vi "SYST_PRES.vi"(0 "VISA IN":refnum<visa-resource-name>, 5 "error in":errorcluster) -> (14 "VISA Out":refnum<visa-resource-name>, 19 "error out":errorcluster)   [LabVIEW 2018, in "PNA-X.lvlib"] (continued)
DISPlay:WINDow<wnum>:TRACe<tnum>TITLe:DATA? \nReturn Type String \nDefault Not Applicable \nDISPlay:WINDow<wnum>:TRACe<tnum>TITLe:STATe <bool> \n(Read-Write) Turns display of the Trace Title ON or OFF. When turned OFF, the previous trace title \nreturns. Set a new trace title using DISP:WIND:TRAC:TITL:DATA \nLearn more about Trace Titles \nParameters \n<wnum> Any existing window number. If unspecified, value is set to 1 \n<tnum> Trace number of the specified window. If unspecified, value is set to 1. The \ntrace number displayed in trace status is the trace number of the channel; not \nthe window. Use Display:Cat? to read the window numbers. Use \nDisp:Window:Cat? to read the trace numbers of the specified window. \n<bool> ON (or 1) - turns the title ON. \nOFF (or 0) - turns the title OFF. \nExamples DISP:WIND:TRAC:TITL ON \nDisplay:window2:trace3:title:state off \nQuery Syntax DISPlay:WINDow<wnum>:TRACe<tnum>:TITLe[:STATe]? \n1598\n\nReturn Type Boolean (1 = ON, 0 = OFF) \nDefault ON \nDISPlay:WINDow<wnum>:TRACe<tnum>:Y[:SCALe]:AUTO \n(Write-only) Performs an Autoscale on the specified trace in the specified window, providing the best \nfit display. Autoscale is performed only when the command is sent; it does NOT keep the trace \nautoscaled indefinitely. \nParameters \n<wnum> Any existing window number. If unspecified, value is set to 1. \n<tnum> Any existing trace number; if unspecified, value is set to 1 \nExamples DISP:WIND:TRAC:Y:AUTO \ndisplay:window2:trace2:y:scale:auto \nQuery Syntax Not applicable \nDefault Not applicable \nDISPlay:WINDow<wnum>:TRACe<tnum>:Y[:SCALe]:PDIVision <num> \n(Read-Write) Sets the Y axis Per Division value of the specified trace in the specified window. \nParameters \n<wnum> Any existing window number. If unspecified, value is set to 1. \n<tnum> Any existing trace number; if unspecified, value is set to 1 \n<num> Units / division value. The range of acceptable values is dependent on format \nand domain. \nNote: This command will accept MIN or MAX instead of a numeric \nparameter. See SCPI Syntax for more information. \nExamples DISP:WIND:TRAC:Y:PDIV 1 \ndisplay:window2:trace2:y:scale:pdivision maximum \nQuery Syntax DISPlay:WINDow<wnum>:TRACe<tnum>:Y[:SCALe]:PDIVision? \nReturn Type Numeric \nDefault 10 \nDISPlay:WINDow<wnum>:TRACe<tnum>:Y[:SCALe]:RLEVel <num> \n1599\n\n(Read-Write) Sets the Y axis Reference Level of the specified trace in the specified window. \nParameters \n<wnum> Any existing window number. If unspecified, value is set to 1. \n<tnum> Any existing trace number; if unspecified, value is set to 1 \n<num> Reference level value. The range of acceptable values is dependent on format \nand domain. \nNote: This command will accept MIN or MAX instead of a numeric parameter. \nSee SCPI Syntax for more information. \nExamples DISP:WIND:TRAC:Y:RLEV 0 \ndisplay:window2:trace2:y:scale:rlevel minimum \nQuery Syntax DISPlay:WINDow<wnum>:TRACe<tnum>:Y[:SCALe]:RLEVel? \nReturn Type Numeric \nDefault NA \nDISPlay:WINDow<wnum>:TRACe<tnum>:Y[:SCALe]:RPOSition <num> \n(Read-Write) Sets the Reference Position of the specified trace in the specified window \nParameters \n<wnum> Any existing window number. If unspecified, value is set to 1. \n<tnum> Any existing trace number; if unspecified, value is set to 1 \n<num> Reference position on the screen measured in horizontal graticules from the \nbottom. The range of acceptable values is dependent on format and domain. \nNote: This command will accept MIN or MAX instead of a numeric \nparameter. See SCPI Syntax for more information. \nExamples DISP:WIND:TRAC:Y:RPOS 0 \ndisplay:window2:trace2:y:rposition maximum \nQuery Syntax DISPlay:WINDow<wnum>:TRACe<tnum>:Y[:SCALe]:RPOSition? \nReturn Type Numeric \nDefault 5 \nDISPlay:VISible <ON | OFF> \n1600\n\n(Read-Write) Makes the PNA application visible or not visible. In the Not Visible state, the analyzer \ncycle time for making measurements, and especially data transfer, can be significantly faster because \nthe display does not process data. \nParameters \n<ON | OFF> ON (or 1) - PNA app is visible \nOFF (or 0) - PNA app is NOT visible \nExamples DISP:VIS ON \ndisplay:visible off \nQuery Syntax DISPlay:VISible? \nReturn Type Boolean (1 = ON, 0 = OFF) \nDefault ON \nLast modified: \n9/12/06 Modified for number of windows. \n1601\n\nFormat Commands \nSpecifies the way that data will be transferred when moving large amounts of data. These commands \nwill affect data that is transferred with the CALC:DATA and CALC:RDATA commands. \nClick on a blue keyword to view the command details. \nSee Also \nExample Programs \nSynchronizing the PNA and Controller \nSCPI Command Tree \nFORMat:BORDer <char> \n(Read-Write) Set the byte order used for GPIB data transfer. Some computers read data from the \nanalyzer in the reverse order. This command is only implemented if FORMAT:DATA is set to \n:REAL. If FORMAT:DATA is set to :ASCII, the swapped command is ignored. \nParameters \n<char> Choose from: \nNORMal - Use when your controller is anything other than an IBM compatible \ncomputers \nSWAPped - for IBM compatible computers \nNote: Use NORMal if you are using drivers like VISA or development \nenvironments like VEE, LabView, or T&M Tool kit. \nExamples FORM:BORD SWAP \nformat:border normal \nQuery Syntax FORMat:BORDer? \nReturn Type Character \n1602\n\nDefault Normal \nFORMat[:DATA] <char> \n(Read-Write) Sets the data format for data transfers. \nTo transfer measurement data, use CALC:DATA. \nTo transfer Cal Set data, use \nTo transfer Source Power correction data, use \nSOURce:POWer:CORRection:COLLect:TABLe:DATA \nSOURce:POWer:CORRection:COLLect:TABLe:FREQuency \nSOURce:POWer:CORRection:DATA \nParameters \n<char> Choose from: \nREAL,32 - (default value for REAL) Best for transferring large amounts of \nmeasurement data. \nREAL,64 - Slower but has more significant digits than REAL,32. Use \nREAL,64 if you have a computer that doesn't support REAL,32. \nASCii,0 - The easiest to implement, but very slow. Use if small amounts of \ndata to transfer. \nNote: The REAL,32 and REAL,64 arguments transfer data in block format as \nexplained in Transferring Measurement Data. \nExamples FORM REAL,64 \nformat:data ascii \nQuery Syntax FORMat:DATA? \nReturn Type Character,Character \nDefault ASCii,0 \n1603\n\nHardcopy Command \nLearn about Printing \nSCPI Command Tree \nHCOPy:FILE <filename> \n(Write-only) Saves the screen image to a file. \nParameters \n<filename> Name of the file to save the screen to. The file is saved to the current working \ndirectory unless a valid full path name is specified. \nUse one of the following suffixes: \n.bmp - not recommended due to large file size \n.jpg - not recommended due to poor quality \n.png - recommended \nExamples HCOPY:FILE \"myFile.png\" \nhcopy:file \"c:\\data\\myfile.png\" \nQuery Syntax Not Applicable \nDefault Not Applicable \nHCOPy[:IMMediate] \n(Write-only) Prints the screen to the default printer. \nExamples HCOP \nhcopy:immediate \nQuery Syntax Not applicable \nDefault Not Applicable \n1604\n\nInitiate Commands \nControls triggering signals \nClick on a blue keyword to view the command details. \nSee Also \nExample Triggering the PNA \nLearn about Triggering \nSynchronizing the PNA and Controller \nSCPI Command Tree \nINITiate:CONTinuous <boolean> \n(Read-Write) Specifies whether the PNA trigger source is set to Internal (continuous) or Manual. \nThis command is a subset of TRIG:SEQ:SOURce, which can also set the trigger source to External. \nTo set how a channel responds to trigger signals, use SENS:SWE:MODE. \nSee a map of user interface to SCPI triggering commands. \nFor more information on triggering, see the PNA Trigger Model. \nSee the Example program: Triggering the PNA using SCPI. \nParameters \n<boolean> ON (or 1) - Internal (continuous) trigger. \nOFF (or 0) - Manual sweep. Use INIT:IMMediate to send a trigger signal \nExamples INIT:CONT ON \ninitiate:continuous off \nQuery Syntax INITiate:CONTinuous? \nReturn Type Boolean (1 = ON, 0 = OFF) \nDefault ON \n1605\n\nINITiate<cnum>[:IMMediate] \n(Write-only) Stops the current sweeps and immediately sends a trigger. (Same as Trigger! on the PNA \nfront panel). \nSee the Example program: Triggering the PNA using SCPI \nNote: An SMC Fixed Output measurement cannot be triggered using this command. For more \ninformation, see the example program. \nThis command requires Trigger:Source to be set to Manual. This causes ONE trigger signal to be \nSENT each time INIT:IMM is issued. \nSens<ch>:Sweep:Mode sets the number of trigger signals each channel will ACCEPT (Continuous - \nunlimited, Groups - a specific number, or HOLD - none.) \nTo trigger ALL channels in turn: \nSet ALL channels to Sens<ch>:Sweep:Mode Continuous. The <ch> argument in INIT<ch>:IMM is \nignored. \nThen�\nTRIG:SCOP ALL triggers ALL channels (in sequence) each time Init:Imm is sent. \nTRIG:SCOP CURRent triggers ONLY the NEXT channel each time Init:Imm is sent. \nTo trigger ONLY a specified channel: \nSet ALL channels to Sens<ch>:Sweep:Mode HOLD 1. \nSend TRIG:SCOP CURRent 2. \nSend Init<ch>:Imm where <ch> is the channel to be triggered. 3. \nAdvanced Situations that require some channels to be in CONT and others in HOLD are rare. The \nfollowing describes the behavior of the Init:Imm command in these situations: \nWhen Trigger:Scope = Global: \nIf the SPECIFIED <cnum> channel is in hold mode, it is put in single trigger (accepts 1 trigger signal) and \ngoes to the end of the queue of channels to be triggered. The other 'non-hold' channels are triggered. The \nnext Init:Imm triggers the specified channel first. \nFor example: ch1 is in Hold, ch2 and ch3 are in CONT and we send INIT1:IMM \n1606\n\nOn the first INIT:IMM, ch2 and ch3 is triggered. \nnext INIT:IMM, ch1, ch2, ch3 is triggered. \nnext INIT:IMM, ch2 and ch3 is triggered. \nnext INIT:IMM, ch1, ch2, ch3 is triggered, and so forth. \nWhen Trigger:Scope = Channel \nOnly ONE channel is triggered for each issued INIT<ch>:IMM command. \nIf the specified channel is in hold, it is put in single trigger (accepts 1 trigger signal) and goes the end of the \nqueue of channels to be triggered as in the 'Global' example. \nThis is one of the PNA overlapped commands. Learn more. \nParameters \n<cnum> Any existing channel number. If unspecified, value is set to 1 \nExamples INIT \ninitiate2:immediate \nQuery Syntax Not applicable \nDefault Not applicable \nLast modified: \nApril 23, 2007 Updated Init:Imm \n1607\n\nMemory Commands \nThe memory commands control saving and loading instrument states and measurement trace data to the \nhard drive. To read and write trace data in GPIB format, see CALC:DATA. \nClick on a blue keyword to view the command details. \nSee Also \nExample Programs \nLearn about Save / Recall and File Types \nSynchronizing the PNA and Controller \nSCPI Command Tree \nSpecifying Path Names \nThe MMEM commands use the following rules to specify path names: \nThe default folder is \"C:\\Program Files\\Agilent\\Network Analyzer\\Documents\" \nYou can change the active directory using MMEMory:CDIRectory. \nSpecify only the file name if using the active directory. \nYou can also use an absolute path name to specify the folder and file. \nMMEMory:CATalog[:<char>]? [<folder>] \n1608\n\n(Read-only) Returns a comma-separated string of file names that are in the specified folder. If there \nare no files of the specified type, \"NO CATALOG\" is returned. Learn about File Types \nParameters \n<char> The type of files to list. Choose from: \nSTATe - Instrument states (.sta) \nCORRection - Calibration Data (.cal) \nCSARchive - Instrument state and calibration data (.csa) \nCSTate - Instrument state and link to Calibration data (.cst) \nIf unspecified then ALL file types (even unknown types) are listed. \n<folder> String - Any existing folder name. See Specifying Path Names \nExamples MMEM:CAT? 'lists all files from the current folder \nmmemory:catalog:correction? 'C:\\Program Files\\Agilent\\Network \nAnalyzer\\Documents' 'lists .cal files from the specified folder \nDefault Not applicable \nMMEMory:CDIRectory <folder> \n(Read-Write) Changes the folder name. \nParameters \n<folder> Any drive and folder name that already exists. \nIf the same level as \"C:\\Program Files\\Agilent\\Network Analyzer\\Documents\", \nthen no punctuation is required \nMMEM:CDIR Service \nIf the new folder is at a different level than \"C:\\Program Files\\Agilent\\Network \nAnalyzer\\Documents\", use a slash (\\) before the folder name and enclose in \nquotes. \nmmemory:cdirectory '\\automation' 'changes default directory up \none level. \nYou can use an absolute path to specify the new folder. \nmmemory:cdirectory 'c:\\automation\\service' \nQuery Syntax MMEMory:CDIRectory? 'Returns the current folder name \n1609\n\nReturn Type String \nDefault 'C:\\Program Files\\Agilent\\Network Analyzer\\Documents' \nMMEMory:COPY <file1>,<file2> \n(Write-only) Copies file1 to file2. Extensions must be specified. \nParameters \n<file1> String - Name of the file to be copied. See Specifying Path Names \n<file2> String - Name of the file to be created from file1. \nExamples MMEM:COPY 'MyFile.cst','YourFile.cst' \nQuery Syntax Not applicable \nDefault Not applicable \nMMEMory:DELete <file> \n(Write-only) Deletes file. Extensions must be specified. \nParameters \n<file> String - Name of the file to be deleted. See Specifying Path Names \nExamples MMEM:DEL 'MyFile.cst' \nQuery Syntax Not applicable \nDefault Not applicable \nMMEMory:LOAD[:<char>] <file> \n1610\n\n(Write-only) Loads the specified file. Learn about File Types \nParameters \n<char> The type of file to load. Choose from: \nSTATe - Instrument states (.sta) \nCORRection - Calibration Data (.cal) \nCSARchive - Instrument state and calibration data (.csa) \nCSTate - Instrument state and link to Calibration data (.cst) \nIf <char> is unspecified, the extension must be included in the filename. \nIf an extension is specified in <file> that does not agree with <char> then no \naction is taken. \n<file> String - Name of the file to be loaded. See Specifying Path Names \nExamples MMEM:LOAD 'MyFile.cst' \nmmemory:load:state 'MyInstState' \nQuery Syntax Not applicable \nDefault Not applicable \nMMEMory:MDIRectory <folder> \n(Write-only) Makes a folder. \nParameters \n<folder> String - Name of the folder to make. See Specifying Path Names \nExamples MMEM:MDIR 'MyFolder' \nmmemory:mdirectory 'c:\\NewFolder' \nQuery Syntax Not applicable \nDefault Not applicable \nMMEMory:MOVE <file1>,<file2> \n1611\n\n(Write-only) Renames <file1> to <file2>. File extensions must be specified. \nParameters \n<file1> String - Name of the file to be renamed. See Specifying Path Names \n<file2> String - Name of the new file. \nExamples MMEM:MOVE 'MyFile.cst','YourFile.cst' \nQuery Syntax Not applicable \nDefault Not applicable \nMMEMory:RDIRectory <folder> \n(Write-only) Removes the specified folder. \nParameters \n<folder> String - Name of the folder to remove. See Specifying Path Names \nExamples MMEM:RDIR 'MyFolder' \nQuery Syntax Not applicable \nDefault Not applicable \nMMEMory:STORe[:<char>] <file> \n(Write-only) Stores the specified file (.sta, .cal, .csa, .cst, prn). \nTo save snp files, use Calc:Data:SNP:PORTs:SAVE. \nTo save *.cti files, use MMEM:STOR:CIT:DATA or MMEM:STOR:CIT:FORM. \nParameters \n<char> The type of file to store. Choose from: \nSTATe - Instrument states (.sta) \nCORRection - Calibration Data (.cal) \nCSARchive - Instrument state and calibration data (.csa) \nCSTate - Instrument state and link to Calibration data (.cst) \nNo <char> is specified for prn. \n1612\n\nIf <char> is unspecified, then the extension must be included in the filename. \nIf an extension is specified in <file> that does not agree with <char> then no \naction is taken. \nLearn about File Types \n<file> String - Name of any valid file that is not already in existence. See Specifying \nPath Names \nExamples MMEM:STOR:STAT 'myState' \nmmemory:store 'c:\\bin\\myState.sta' \nMMEM:STOR 'MyData.prn' \nQuery Syntax Not applicable \nDefault Not applicable \nMMEMory:STORe:CITifile:DATA <filename> \n(Write only) Saves UNFORMATTED trace data to .cti file. Learn more. \nParameters \n<filename> Any drive and folder name that already exists. \nIf the same level as \"C:\\Program Files\\Agilent\\Network Analyzer\\Documents\", \nthen no punctuation is required \nMMEM:STOR:CIT:DATA MYCTIFile \nIf the new folder is at a different level than \"C:\\Program Files\\Agilent\\Network \nAnalyzer\\Documents\", use a slash (\\) before the folder name and enclose in \nquotes. \nmmemory:cdirectory '\\automation' 'changes default directory up \none level. \nYou can use an absolute path to specify the new folder. \nmmemory:cdirectory 'c:\\automation\\service' \nQuery Syntax Not Applicable \nDefault C:\\Program Files\\Agilent\\Network Analyzer\\Documents' \nMMEMory:STORe:CITifile:FORMat <filename> \n1613\n\n(Write only) Saves FORMATTED trace data to .cti file. Learn more. \nParameters \n<filename> Any drive and folder name that already exists. \nIf the same level as \"C:\\Program Files\\Agilent\\Network Analyzer\\Documents\", \nthen no punctuation is required \nMMEM:STOR:CIT:DATA MYFile \nIf the new folder is at a different level than \"C:\\Program Files\\Agilent\\Network \nAnalyzer\\Documents\", use a slash (\\) before the folder name and enclose in \nquotes. \nmmemory:cdirectory '\\automation' 'changes default directory up \none level. \nYou can use an absolute path to specify the new folder. \nmmemory:cdirectory 'c:\\automation\\service' \nQuery Syntax Not Applicable \nDefault C:\\Program Files\\Agilent\\Network Analyzer\\Documents' \nMMEMory:STORe:TRACe:CONTents:CITifile <char> \n(Read-Write) Specifies the contents of subsequent citifile save statements. (See Data Define Saves) \nParameters \n<char> Choose from: \nSING - Single trace \nDISP - All displayed traces \nAUTO - All displayed traces \nExamples MMEM:STOR:TRAC:CONT:CIT SING \nQuery Syntax MMEMory:STORe:TRACe:CONTents? \nReturn Type Character \nDefault Auto \nMMEMory:STORe:TRACe:FORMat:CITifile <char> \n1614\n\n(Read-Write) Specifies the format of subsequent citifile save statements. (See Data Define Saves) \nParameters \n<char> Format in which the citifile will be saved with subsequent \nMMEMory:STORe:CIT:FORMat statements. Choose from: \nMA - Linear Magnitude / degrees \nDB - Log Magnitude / degrees \nRI - Real / Imaginary \nAUTO - Format in which the trace is already displayed. If other than Log \nMag, Linear Magnitude, or Real/Imag, then the format will be in Real/Imag. \nExamples MMEM:STOR:TRAC:FORM:CIT MA \nQuery Syntax MMEMory:STORe:TRACe:FORMat:CITifile? \nReturn Type Character \nDefault Auto' \nMMEMory:STORe:TRACe:FORMat:SNP <char> \n(Read-Write) Specifies the format of subsequent .s1p, .s2p, .s3p; s4p save statements. (See Data \nDefine Saves). \nParameters \n<char> Choose from: \nMA - Linear Magnitude / degrees \nDB - Log Magnitude / degrees \nRI - Real / Imaginary \nAUTO - data is output in currently selected trace format. If other than LogMag, \nLinMag, or Real/Imag, then output is in Real/Imag. \nExamples MMEM:STOR:TRAC:FORM:SNP MA \nQuery Syntax MMEMory:STORe:TRACe:FORMat:SNP? \nReturn Type Character \nDefault Auto' \n1615\n\nMMEMory:TRANsfer <fileName>,<dataBlock> \n(Read-Write) Transfers data between the PNA and an external controller. Other MMEM commands \ntransfer data between the PNA application and the PNA hard drive. If <fileName> already exists, it \nwill be overwritten. The file must be no larger than 20MB. \nTo read trace data from the PNA in block format, use CALC:DATA. \nParameters \n<fileName> String - File name. See Specifying Path Names \n<dataBlock> Block Data - The contents of the file. \nThe data block is a block of binary data. Use the following syntax: \n#<num digits><byte count><data bytes><NL><END> \nwhere: \n<num_digits> specifies how many digits are contained in <byte_count> \n<byte_count> specifies how many data bytes will follow in <data bytes> \nExample See example program \nQuery Syntax MMEMory:TRANsfer? <fileName> \nReads block data from the specified file location. \nDefault Not applicable \nLast modified: \n9/12/06 MQ Store command has reference to PORTS Snp. \n1616\n\nOutput Command \nLearn about Power \nOUTPut[:STATe] <ON | OFF> \n(Read-Write) Turns RF power from the source ON or OFF. \nSee note about source power state with instrument state save and recall. \nParameters \n<ON | OFF> ON (or 1) - turns RF power ON \nOFF (or 0) - turns RF power OFF \nExamples OUTP ON \noutput:state off \nQuery Syntax OUTPut[:STATe]? \nReturn Type Boolean (1 = ON, 0 = OFF) \nDefault ON \n1617\n\nRoute Command \nLearn about Frequency Offset \nSCPI Command Tree \nROUTe<cnum>:PATH:LOOP[:R1] <char> \n(Read-Write) Throws internal switch to reference receiver when the specified channel is measured. \nThis feature is only available on PNA models with Option 081 - external reference switch. See block \ndiagram of the reference switch. \nParameters \n<cnum> Any existing channel number. If unspecified, value is set to 1 \n<char> Position of the switch. Choose from: \nINTernal - bypass R1 Loop. Connects the port 1 source directly to the R1 \nreceiver. \nEXTernal - flow through R1 Loop. Allows direct access to the R1 receiver \nthrough the Reference 1 front-panel connectors. \nExamples ROUT:PATH:LOOP INT \nroute2:path:loop:r1 external \nQuery Syntax ROUTe<cnum>:PATH:LOOP:R1? \nReturn Type Character \nDefault INTernal \n1618\n\nSense:Average Commands \nSets sweep-to-sweep averaging parameters. Averaging is a noise reduction technique that averages \neach data point over a user-specified number of sweeps. Averaging affects all of the measurements in \nthe channel. \nClick on a blue keyword to view the command details. \nSee Also \nExample using some of these commands. \nLearn about Averaging \nSynchronizing the PNA and Controller \nSCPI Command Tree \nSENSe<cnum>:AVERage:CLEar \n(Write-only) Clears and restarts averaging of the measurement data. Must also set \nSENS:AVER[:STATe] ON \nParameters \n<cnum> Any existing channel number; if unspecified, value is set to 1. \nExamples SENS:AVER:CLE \nsense2:average:clear \nQuery Syntax Not applicable \nDefault Not applicable \nSENSe<cnum>:AVERage:COUNt <num> \n1619\n\n(Read-Write) Sets the number of measurement sweeps to combine for an average. Must also set \nSENS:AVER[:STATe] ON \nParameters \n<cnum> Any existing channel number; if unspecified, value is set to 1. \n<num> Number of measurement sweeps to average. Choose any number between 1 \nand 65536 (2^16). \nExamples SENS:AVER:COUN 999 \nsense2:average:count 73 \nQuery Syntax SENSe<cnum>:AVERage:COUNt? \nReturn Type Numeric \nDefault 1 \nSENSe<cnum>:AVERage[:STATe] <ON | OFF> \n(Read-Write) Turns trace averaging ON or OFF. \nParameters \n<cnum> Any existing channel number; if unspecified, value is set to 1. \n<ON | OFF> ON (or 1) - turns averaging ON. \nOFF (or 0) - turns averaging OFF. \nExamples SENS:AVER ON \nsense2:average:state off \nQuery Syntax SENSe<cnum>:AVERage[:STATe]? \nReturn Type Boolean (1 = ON, 0 = OFF) \nDefault Off \n1620\n\nSense:Bandwidth Commands \nSee Also \nExample Programs \nLearn about IF Bandwidth \nSynchronizing the PNA and Controller \nSCPI Command Tree \nSENSe<cnum>:BANDwidth | BWIDth[:RESolution] <num> \n(Read-Write) Sets the bandwidth of the digital IF filter to be used in the measurement. (Use either \nSense:Bandwidth or Sense:Bwidth) \nParameters \n<cnum> Any existing channel number. If unspecified, value is set to 1 \n<num> IF Bandwidth in Hz. The list of valid IF Bandwidths is different depending on \nthe PNA model. (Click to see the lists.) If an invalid number is specified, the \nanalyzer will round up to the closest valid number. \nExamples SENS:BWID 1KHZ \nsense2:bandwidth:resolution 1000 \nQuery Syntax SENSe<cnum>:BANDwidth | BWIDth[:RESolution]? \nReturn Type Numeric \nDefault See Preset IFBW for your PNA model. \nSENSe<cnum>:BANDwidth | BWIDth:TRACk <bool> \n1621\n\n(Read-Write) Sets and returns the state of the Reduce IF BW at Low Frequencies feature. \n(Use either Sense:Bandwidth:Track or Sense:Bwidth:Track). \nParameters \n<cnum> Any existing channel number. If unspecified, value is set to 1 \n<bool> Choose from: \nON or 1 - Reduce IF BW at Low Frequencies is set ON \nOFF or 0 - Reduce IF BW at Low Frequencies is set OFF \nExamples SENS:BWID:TRAC OFF \nsense2:bandwidth:track 1 \nQuery Syntax SENSe<cnum>:BANDwidth | BWIDth:TRACk? \nReturn Type Boolean \nDefault ON \n1622\n\nSense:Correction Commands \nPerforms and applies calibration and other error correction features. \nTo perform Guided Calibration, see Sens:Corr Coll:GUIDed. \n1623\n\nClick on a blue keyword to view the command details. \nSee Also \nExample Programs \nNew See Calibrating the PNA Using SCPI \nLearn about Measurement Calibration \nSynchronizing the PNA and Controller \nSCPI Command Tree \nSENSe<cnum>:CORRection:CCHeck[:ACQuire] <mod>[,char] \n(Write-only) Reads the 'confidence data' associated with the specified ECal module and puts it into \nmemory. The measurement is selected using SENS:CORR:CCH:PAR. This command is compatible \nwith *OPC. \nParameters \n<cnum> Any existing channel number. If unspecified, value is set to 1. \n<mod> ECAL Module that contains the confidence data. Choose from: \nECAL1 \n..through.. \nECAL8 \n[char] Optional argument. Specifies which characterization within the ECal module \nthat the confidence data will be read from. \nCHAR0 Factory characterization (data that was stored in the ECal module by \n1624\n\nAgilent). Default if not specified. \nCHAR1 User characterization #1 \nCHAR2 User characterization #2 \nCHAR3 User characterization #3 \nCHAR4 User characterization #4 \nCHAR5 User characterization #5 \nExamples SENS:CORR:CCHeck ECAL2 \nsense2:correction:ccheck:acquire ecal1,char1 \nQuery Syntax Not applicable \nDefault Not applicable \nSENSe<cnum>:CORRection:CCHeck:DONE \n(Write-only) Concludes the Confidence Check and sets the ECal module back into the idle state. \nParameters \n<cnum> Any existing channel number. If unspecified, value is set to 1 \nExamples SENS:CORR:CCH:DONE \nsense2:correction:ccheck:done \nQuery Syntax Not applicable \nDefault Not applicable \nSENSe<cnum>:CORRection:CCHeck:PARameter <Mname> \n1625\n\n(Read-Write) Specifies an existing measurement to be used for the Confidence Check. \nParameters \n<cnum> Any existing channel number. If unspecified, value is set to 1 \n<Mname> Name of the measurement you are selecting for the confidence check. The \nmeasurement must already exist. \nExamples SENS:CORR:CCH:PAR 'TEST' \n'selects the measurement \"test\" on channel 1 for the confidence \ncheck \nsense2:correction:ccheck:parameter 'test' \n'selects the measurement \"test\" on channel 2 for the confidence \ncheck \nQuery Syntax SENSe<cnum>:CORRection:CCHeck:PARameter? \nReturns the name of the selected measurement on channel <cnum>. \nReturn Type String \nDefault Not applicable \nSENSe<cnum>:CORRection:COLLect[:ACQuire] <class>[,subclass] \n(Write-only) For UNGUIDED calibration, measures the specified standards from the selected \ncalibration kit. The calibration kit is selected using the Sense:Correction:Collect:CKIT command. \nFor using two sets of standards, see SENS:CORR:TST. \nNote: Before using this command you must select two items: \n1. Select a calibration method using SENS:CORR:COLL:METH \n2. Select a measurement using CALC:PAR:SEL. You can select one measurement for each channel. \nParameters \n<cnum> Any existing channel number. If unspecified, value is set to 1 \n<class> Measures the standards associated with these class labels. Choose from: \n1626\n\nLabel Forward Reverse \nSTAN1 S11A S22A \nSTAN2 S11B S22B \nSTAN3 S11C S22C \nSTAN4 S21T S12T \nSTAN5 Generic Isolation; not associated with calibration kit definition. \nECAL1 \nthrough \nECAL8 \nECAL modules \nPOWer Take a receiver power cal sweep and turn correction ON \nSLSET Sets 'sliding load type', and increments the \"number of slides\" count. \nThe total number of slides is critical to the correct calculation of the \nsliding load algorithm. See a sliding load cal example. \nSLDONE Computes the sliding load using a circle fit algorithm. \n[subclass] Optional argument. For mechanical calibration kits, choose from the following to \nspecify the standard to be acquired from the SENS:CORR:COLL:CKIT:ORDer list. \nIf not specified, subclass is set to SST1. \nSST1 First standard in the order list \nSST2 Second standard in the order list \nSST3 Third standard in the order list \nSST4 Fourth standard in the order list \nSST5 Fifth standard in the order list \nSST6 Sixth standard in the order list \nSST7 Seventh standard in the order list \nIf an ECAL module (1 through 8) is specified for <class>, choose one of the \nfollowing for specifying which characterization within the ECal module will be \nused for the acquire. If not specified, the default is CHAR0. \nCHAR0 Factory characterization (data that was stored in the ECal module by \nAgilent) \nCHAR1 User characterization #1 \nCHAR2 User characterization #2 \nCHAR3 User characterization #3 \nCHAR4 User characterization #4 \nCHAR5 User characterization #5 \n1627\n\nExamples SENS:CORR:COLL STAN1 \n'If SENS:CORR:COLL:CKIT:ORDer2 5,3,7 \nwas specified, the following command measures standard 3 (the \nsecond in the order list) \nsense1:correction:collect:acquire stan3,sst2 \nSENS:CORR:COLL ECAL4 \nsense2:correction:collect:acquire ecal2,char1 \nQuery Syntax Not applicable \nDefault Not applicable \nSENSe<cnum>:CORRection:COLLect:APPLy \n(Write-only) Applies error terms to the measurement that is selected using Calc:Par:Select. \nNote: Before using this command you must select a measurement using CALC:PAR:SEL. You can \nselect one measurement for each channel. \nNote: This command is only necessary if you need to modify error terms. If you do not need to modify \nerror terms, SENSe<cnum>:CORRection:COLLect:SAVE calculates and then automatically applies \nerror terms after you use SENS:CORR:COLL:ACQuire to measure cal standards. \nParameters \n<cnum> Any existing channel number. If unspecified, value is set to 1 \nExample CALCulate2:PARameter:SELect S21_2 'select the measurement to \napply terms to \n1. \nSENSe2:CORRection:COLLect:METHod SPARSOLT 'set type of cal \nmethod. \n2. \nCALCulate2:DATA? SCORR1 'download the error term of interest 3. \n'Modify the error term here 4. \nCALCulate2:DATA SCORR1 'upload the error term of interest 5. \nSENSe2:CORRection:COLLect:APPLy 'applies the error terms to \nthe measurement \n6. \nQuery Syntax Not applicable \nDefault Not applicable \n1628\n\nSENSe:CORRection:COLLect:ISOLation:AVERage:INCRement <num> \n(Read-Write) Specifies amount to increment (increase) the channel averaging factor during isolation \nmeasurement of the ECal module during an unguided ECal calibration. \nNote: if the channel currently has averaging turned OFF and <num> is greater than 1, averaging will \nbe turned ON only during the isolation measurements and with the averaging factor equal to <num>. \nParameters \n<num> Incremental Averaging factor. The maximum averaging factor is 65536 (2^16). \nExamples SENS:CORR:COLL:ISOL:AVER:INCR 16 \nsense:correction:collect:isolation:average:increment 0 \nQuery Syntax SENSe:CORRection:COLLect:ISOLation:AVERage:INCRement? \nReturn Type Numeric \nDefault 8 - If this command is NOT sent, but ECal isolation is measured, then \naveraging will be turned ON with factor set to 8 during the isolation \nmeasurement. \nSENSe<cnum>:CORRection:COLLect:ISOLation:ECAL:[:STATe] <bool> \n(Read-Write) Specifies whether or not the isolation state of the ECal module will be measured as part \nof an unguided ECal calibration. \nAn unguided calibration is performed using the SENS:CORR:COLL:METH and \nSENS:CORR:COLL:ACQ commands. \nNote: The inherent isolation of the PNA is better than that attained with this command. ONLY use \nthis command when using an external test set, and ONLY using a 8509x ECal module. \nParameters \n<cnum> Any existing channel number. If unspecified, value is set to 1 \n<bool> ON (or 1) - isolation is measured during the unguided ECal calibration. \nOFF (or 0) isolation is NOT measured during the unguided ECal calibration. \nExamples SENS1:CORR:COLL:ISOL:ECAL ON \nsense2:correction:collect:isolation:ecal:state 0 \nQuery Syntax SENSe:CORRection:COLLect:ISOLation:ECAL:STATe? \nReturn Type Boolean (1 = ON, 0 = OFF) \nDefault OFF \n1629\n\nSENSe<cnum>:CORRection:COLLect:METHod <char> \n(Read-Write) For UNGUIDED calibration, sets the calibration method (also known as 'Calibration \nType' on calibration dialog box.) To select a Cal Type from a Cal Set, use CALC:CORR:TYPE. \nNote: Before using this command you must select a measurement using CALC:PAR:SEL. You can \nselect one measurement for each channel. \nParameters \n<cnum> Any existing channel number. If unspecified, value is set to 1 \n<char> Choose from: \nMethod Description \nNONE No Cal method \nREFL1OPEN Response Open \nREFL1SHORT or \nREFL1 \nResponse Short \nREFL3 Full 1 port \nRPOWer Receiver Power Cal \nTRAN1 Response Thru \nTRAN2 Response Thru and Isolation \nSPARSOLT Full SOLT 2 port \nSPARTRL TRL Cal (not available on all PNAs.) \nExamples SENS:CORR:COLL:METH REFL1 \nsense2:correction:collect:method sparsolt \nQuery Syntax SENSe<cnum>:CORRection:COLLect:METHod? \nReturn Type Character \nDefault Not Applicable \nSENSe<cnum>:CORRection:COLLect:SAVE \n1630\n\n(Write-only) For UNGUIDED calibrations ONLY. This command does the following: \ncalculates the error terms using the selected :METHod, \napplies the error terms to the selected measurement (turns error correction ON.) \nsaves the calibration error-terms to the channels Cal Register or a User Cal Set. \nThe Cal Register or User Cal Set is determined by the setting of the \nSENS:CORR:PREFerence:CSET:SAVE command. \nDo NOT use this command during an ECAL. When performing an ECAL calibration using \nSENS:CORR:COLL:ACQuire, this SAVE operation is performed automatically before the \ncompletion of a successful ACQuire. \nBefore using this command you must select a measurement using CALC:PAR:SEL. You can select \none measurement for each channel. \nParameters \n<cnum> Any existing channel number. If unspecified, value is set to 1 \nExamples SENS:CORR:COLL:SAVE \nsense2:correction:collect:save \nQuery Syntax Not applicable \nDefault Not applicable \nSENSe:CORRection:IMPedance:INPut:MAGNitude <num> \n(Read-Write) Sets and returns the system impedance value for the analyzer. \nParameters \n<num> System Impedance value in ohms. Choose any number between 0 and 1000 \nohms. \nExamples SENS:CORR:IMP:INP:MAGN 75 \nsense:correction:impedance:input:magnitude 50.5 \nQuery Syntax SENSe:CORRection:IMPedance: \nINPut:MAGNitude? \nReturn Type Numeric \nDefault 50 \n1631\n\nSENSe<cnum>:CORRection:INTerpolate[:STATe] <ON | OFF> \n(Read-Write) Turns correction interpolation ON or OFF. \nNote: Before using this command you must select a measurement using CALC:PAR:SEL. You can \nselect one measurement for each channel. \nParameters \n<cnum> Any existing channel number. If unspecified, value is set to 1 \n<ON | OFF> ON (or 1) - turns interpolation ON. \nOFF (or 0) - turns interpolation OFF. \nExamples SENS:CORR:INT ON \nsense2:correction:interpolate:state off \nQuery Syntax SENSe<cnum>:CORRection:INTerpolate[:STATe]? \nReturn Type Boolean (1 = ON, 0 = OFF) \nDefault ON \nSENSe<cnum>:CORRection:ISOLation[:STATe] <ON | OFF> OBSOLETE \nThis command no longer works beginning in the PNA 5.2 release. To perform isolation as part of an \nunguided calibration, you must explicitly measure the isolation standard using \nSENS:CORR:COLL:ACQ Stan5. See Example program. \nTo measure isolation as part of an ECal, use SENS:CORR:COLL:ISOL:ECAL. \n(Read-Write) Turns isolation cal ON or OFF during Full 2-port calibration. If this command is not \nsent, the default state is to disable Isolation. \nParameters \n<cnum> Any existing channel number. If unspecified, value is set to 1 \n<ON | OFF> ON (or 1) - turns isolation ON. \nOFF (or 0) - turns isolation OFF. \nExamples SENS:CORR:ISOL ON \nsense2:correction:isolation:state off \nQuery Syntax SENSe<cnum>:CORRection:ISOLation[:STATe]? \nReturn Type Boolean (1 = ON, 0 = OFF) \nDefault OFF - (Isolation disabled) \nSENSe:CORRection:PREFerence:CSET:SAVE <char> \n1632\n\nImportant Notes: \nThis command replaces SENS:CORR:PREF:CSET:SAVU \nWith 6.0 we implemented a change that defaults to saving completed calibrations to Cal Registers instead \nof User Cal Sets. To revert to the old behavior, send this command with the USER argument. \n(Read-Write) Specifies the default manner in which calibrations that are performed using SCPI or \nCOM are to be stored. Cal data is ALWAYS stored to the channel Cal Register regardless of this \nsetting. \nThis setting survives instrument preset and reboot. It remains until changed by another execution of \nthis command. \nNote: Cal Set arguments used with commands such as SENS:CORR:COLL:GUID:INIT, \nSENS:CORR:COLL:GUID:SAVE and SENS:CORR:COLL:GUID:SAVE:CSET will override of any \nof these default preference settings. \nLearn about Cal Registers and User Cal Sets. \nParameters \n<char> CALRegister - Cal is saved ONLY to the channel Cal Register. \nUSER - Cal is saved to a new User Cal Set file when performing a SCPI \ncalibration. The Cal Set name is automatically generated. To change the name, \nsend SENS:CORR:CSET:NAME after the cal is complete. This reverts to pre- \n6.0 behavior. \nREUSe - The cal is saved to the Cal Set that is currently selected on the \nspecified channel, which could be the channel Cal Register. If the channel does \nnot yet have a selected Cal Set, the cal will be saved to a new User Cal Set with \nan automatically-generated name. \nExamples SENS:CORR:PREF:CSET:SAVE USER \nsense:correction:preference:cset:save reuse \nQuery Syntax SENSe:CORRection:PREFerence:CSET:SAVE? \nReturn Type Character \nDefault CALRegister \nSENSe:CORRection:PREFerence:CSET:SAVUser <bool> Superseded \n1633\n\nThis command is replace with SENS:CORR:PREF:CSET:SAVE \nNOTE: With 6.0 we implemented a change that defaults to saving completed calibrations to Cal \nRegisters instead of User Cal Sets. To revert to the old behavior, send this command as ON (1). For \nUI and COM use, this can be done from the GPIB console. \n(Read-Write) Specifies whether cal data is automatically saved to a User Cal Set file after performing \na SCPI calibration. Cal data is always saved to a Cal Register regardless of this setting. \nThis setting survives instrument preset and reboot. It remains until changed by another execution of \nthis command. \nLearn about Cal Registers and User Cal Sets. \nParameters \n<bool> ON or 1 - Cal is automatically saved to a User Cal Set file when performing a \nSCPI calibration. The Cal Set name is automatically generated. To change the \nname, send SENS:CORR:CSET:NAME after the cal is complete. Reverts to \npre-6.0 behavior. \nOFF or 0 - Cal is NOT automatically saved to a User Cal Set. To save a \ncalibration to a User Cal Set, use SENS:CORR:COLL:GUID:INIT. \nExamples SENS:CORR:PREF:CSET:SAVU 1 \nsense:correction:preference:cset:savuser 0 \nQuery Syntax SENSe:CORRection:PREFerence:CSET:SAVUser? \nReturn Type Boolean (1 = ON, 0 = OFF) \nDefault OFF (0) \nSENSe:CORRection:PREFerence:ECAL:ORIentation[:STATe] <ON|OFF> \n1634\n\n(Read-Write) Specifies whether or not the PNA should perform orientation of the ECal module \nduring calibration. Orientation is a technique by which the PNA automatically determines which \nports of the module are connected to which ports of the PNA. Orientation begins to fail at very low \npower levels or if there is much attenuation in the path between the PNA and the ECal module. If \norientation is turned OFF, the SENS:CORR:PREF:ECAL:PMAP command must be used to specify \nthe port connections before performing a cal. \nNote: For 3-port or 4-port measurements, when orientation is OFF, you are not allowed to specify \nhow the ECAL module is connected. Instead, the PNA determines the orientation. Use \nSENS:CORR:COLL:GUID:DESC? to query the orientation. The PNA does not verify that you made \nthe connection properly. \nThis setting remains until the PNA is restarted or this command is sent again. \nParameters \n<bool> ECAL orientation state. Choose from: \nON or 1 - PNA performs orientation of the ECal module. \nOFF or 0 - PNA does NOT performs orientation of the ECal module. \nExamples SENS:CORR:PREF:ECAL:ORI OFF \nsense:correction:preference:ecal:orientation:state on \nQuery Syntax SENSe:CORRection:PREFerence:ECAL:ORIentation[:STATe]? \nReturn Type Boolean (1 = ON, 0 = OFF) \nDefault ON (1) \nSENSe:CORRection:PREFerence:ECAL:PMAP <module>,<string> \n(Read-Write) When ECal module orientation is turned OFF (SENS:CORR:PREF:ECAL:ORI), this \ncommand specifies the port mapping (which ports of the module are connected to which ports of the \nPNA) prior to performing ECal calibrations. \nThis setting remains until the PNA is restarted or this command is sent again. \nParameters \n<module> Specifies which ECal module this port map is being applied to. Choose from: \nECAL1 \n.through. \nECAL8 \n1635\n\n<string> Format this parameter in the following manner: \nAw,Bx,Cy,Dz \nwhere\nA, B, C, and D are literal ports on the ECAL module \nw,x,y, and z are substituted for PNA port numbers to which the ECAL module port \nis connected. \nPorts of the module which are not used are omitted from the string. \nFor example, on a 4-port ECal module with \nport A connected to PNA port 2 \nport B connected to PNA port 3 \nport C not connected \nport D connected to PNA port 1 \nthe string would be: A2,B3,D1 \nIf either the receive port or source port (or load port for 2-port cal) of the \nCALC:PAR:SELected measurement is not in this string and orientation is OFF, \nan attempt to perform an ECal calibration will fail. \nExamples SENS:CORR:PREF:ECAL:PMAP ECAL2, 'A1,B2' \nsense:correction:preference:ecal:pmap ecal3, 'a2,b1,c3' \nQuery Syntax SENSe:CORRection:PREFerence:ECAL:PMAP? <module> \nReturn Type String \nDefault Null string () \nSENSe:CORRection:PREFerence:SIMCal <bool> \n1636\n\n(Read-Write) Sets and returns a preference for the Unguided Cal behavior described below. This \nsetting persists until it is changed. \nThis preference can also be set True by executing the script on the PNA at C:/Program \nFiles/Agilent/Network Analyzer/System/wincal32.reg. \nParameters \n<bool> Boolean - Choose from: \n0 - False - Reverts to new (preferred) behavior. An error is returned if standard \ndata is not acquired before sending SENS:CORR:COLL:SAVE. \n1 - True - (WinCal compatible) Prevents SENS:CORR:COLL:SAVE from \nfailing when standard data has not, and will not, be acquired. \nLearn more about old and new behaviors. \nExamples SENS:CORR:PREF:SIMC 0 \nsense:correction:preference:simcal 1 \nQuery Syntax SENSe:CORRection:PREFerence:SIMCal? \nReturn Type Boolean \nDefault 0 \nSENSe:CORRection:PREFerence:TRIG:FREE <char>, <bool> \n(Read-Write) Sets and returns the preference for the trigger behavior during a calibration. This setting \npersists until it is changed. \nNote: If TRIGger:SOURce = Manual, during a calibration the PNA ALWAYS switches to Internal for \none trigger, then back to Manual, regardless of this preference command. \nParameters \n<char> Character - Calibration type. Choose from: \nGUIDed - preference setting pertains to a Guided calibration. \nUNGuided - preference setting pertains to an Unguided calibration. \n<bool> Boolean - Choose from: \n0 - False - The trigger behavior during the specified calibration type DOES \nrespect the setting of the TRIGger:SOURce command. For example,when \nTrigger source = External, the single trigger method will wait for the External \n1637\n\ntrigger signal and then allow only one sweep. \n1 - True - (Pre-6.0 behavior) The trigger behavior during the specified \ncalibration type does NOT respect the setting of the TRIGger:SOURce \ncommand. For example, when Trigger source = External, during calibration the \nPNA switches to Internal sweep, responds to one trigger signal to measure the \nstandard, then switches back to External. \nExamples SENS:CORR:PREF:TRIG:FREE GUID,1 \nsense:correction:preference:trig:free unguided,0 \nQuery Syntax SENSe:CORRection:PREFerence:TRIG:FREE? <char> \nReturn Type Boolean \nDefault False for both calibration types. \nSENSe<cnum>:CORRection:RPOWer:OFFSet[:AMPLitude] <num> \n(Read-Write) Adjusts a receiver power cal to account for components or adapters that are added \nbetween the source port and receiver while performing this cal. For more information, see Receiver \nCal. \nParameters \n<cnum> Any existing channel number. If unspecified, value is set to 1 \n<num> Offset Value in dB. Specify loss as a negative number; and gain as a positive \nnumber. Choose a number between -200 and 200. \nExamples SENS:CORR:RPOW:OFFS .5 \nsense2:correction:rpower:offset:amplitude .-5 \nQuery Syntax SENSe<cnum>:CORRection:RPOWer:OFFSet[:AMPLitude]? \nReturn Type Numeric \nDefault 0 \nSENSe<cnum>:CORRection:RVELocity:COAX <num> \n1638\n\n(Read-Write) Sets the velocity factor to be used with Electrical Delay and Port Extensions. \nParameters \n<cnum> Any existing channel number. If unspecified, value is set to 1 \n<num> Velocity factor. Choose a number between 0 and 10 \n(.66 polyethylene dielectric; .7 teflon dielectric) \nExamples SENS:CORR:RVEL:COAX .66 \nsense2:correction:rvelocity:coax .70 \nQuery Syntax SENSe<cnum>:CORRection:RVELocity:COAX? \nReturn Type Numeric \nDefault 1 \nSENSe:CORRection:SFORward[:STATe] <boolean> \n(Read-Write) Sets the direction a calibration will be performed when only one set of standards is used. \nUse SENSe:CORRection:TSTandards[:STATe] OFF to specify that only one set of standards will be \nused. \nParameters \n<boolean> ON (1) - FORWARD direction of a 2-port calibration will be performed \nOFF (0) - REVERSE direction of a 2-port calibration will be performed \nExamples SENS:CORR:SFOR 1 \nsense:correction:sforward:state 0 \nSee an example using this command \nQuery Syntax SENSe:CORRection:SFORward[:STATe]? \nReturn Type Boolean \nDefault ON \nSENSe<cnum>:CORRection[:STATe] <ON | OFF> \n1639\n\n(Read-Write) Turns error correction ON and OFF for the specified channel. \nNote: Before using this command you must select a measurement using CALC:PAR:SEL. You can \nselect one measurement for each channel. \nParameters \n<cnum> Any existing channel number. If unspecified, value is set to 1 \n<ON | OFF> ON (or 1) - correction is applied to the channel. \nOFF (or 0) - correction is NOT applied to the channel. \nExamples SENS:CORR ON \nsense2:correction:state off \nQuery Syntax SENSe<cnum>:CORRection[:STATe]? \nTo query the error correction state for a measurement, use CALC:CORR:STATe? \nReturn Type Boolean (1 = ON, 0 = OFF) \nDefault OFF \nSENSe:CORRection:TSTandards[:STATe] <boolean> \n(Read-Write) Specifies the acquisition of calibration data using ONE or TWO sets of standards. \nParameters \n<boolean> ON (1) - TWO identical sets of standards will be used to simultaneously \ncalibrate two ports (for both Forward and Reverse parameters). \nOFF (0)- ONE set of standards will be used to perform a full 2-port calibration, \none port at a time. \nWhen specifying ON (use two sets), the SENS:CORR:COLL:ACQuire \ncommand uses the same standard index for each calibration class. To specify \nthe calibration standard gender for each port, you must first ensure that the \norder of calibration class accurately reflects the configuration of your DUT. \nFor example, for a DUT with a male connector on port 1 and a female \nconnector on port 2, order the devices within the S11 classes (A, B, and C) \nsuch that the MALE standards are first in the list. Then order the S22 classes \nspecifying the FEMALE standards as the first in the list. \nExamples SENS:CORR:TST 1 \nsense:correction:tstandard:state 0 \nSee an example using this command \n1640\n\nQuery Syntax SENSe:CORRection:TSTandards[:STATe]? \nReturn Type Boolean \nDefault ON \nSENSe:CORRection:TYPE:CATalog? <char> \n(Read-Write) Lists the Cal Types in the PNA by either GUID or registered name. Learn more about \napplying Cal Type using SCPI. \nNote: Before using this command you must select a measurement using CALC:PAR:SEL. You can \nselect one measurement for each channel. \nParameters \n<char> Specifies the type of list. Choose from: \nGUID - the registered GUID of the Cal Type \nNAME - the registered name of the Cal Type \nExamples SENS:CORR:TYPE:CAT? GUID \nQuery Syntax SENSe<cnum>:CORRection:TYPE:CATalog? <char> \nReturn Type Comma-separated string \nDefault Not Applicable \nLast modified: \nApril 14, \n2007 \nAddd ECal isolation commands \nOct 30, \n2006 \nModified SavUser command \n1641\n\nSense:Correction:Collect:Guided Commands \nPerforms and applies a SmartCal (Guided) calibration and other error correction features. \nClick on a blue keyword to view the command details. \nSee Also \nExamples using these commands. \n1642\n\nNew Calibrating the PNA Using SCPI \nLearn about Measurement Calibration \nSynchronizing the PNA and Controller \nSENSe:CORRection:COLLect:GUIDed:ACQuire <std> \n(Write-only) Initiates the measurement of the specified calibration standard. Executing this command \nwith an unnecessary standard has no affect. \nThe measured data is stored and used for subsequent calculations of error correction coefficients. All \nstandards must be measured before a calibration can be completed. Any measurement can be repeated \nuntil the SENS:CORR:COLL:GUID:SAVE command is executed. \nQuery the user prompt description using SENS:CORR:COLL:GUID:DESC? \nQuery the required calibration steps using SENS:CORR:COLL:GUID:STEP? \nParameters \n<cnum> Any existing channel number. If unspecified, value is set to 1 \n<std> Choose from:STAN1, STAN2, STAN3, through STAN40 \nExamples SENS:CORR:COLL:GUID:ACQ STAN1 \nsense:correction:collect:guided:acquire stan1 \nQuery Syntax Not Applicable \nDefault Not Applicable \nSENSe<cnum>:CORRection:COLLect:GUIDed:ADAPter:CREate? <conn1>, <conn2> \n(Read-only) Specifies the use of a THRU adapter to be used during the Guided Cal Unknown THRU \nand Adapter Removal Cal. Returns an adapter index <n> which is used to refer to the adapter in \nseveral related commands. See Cal Thru Methods. While the choice of which end of the adapter is \n<conn1> and <conn2> is arbitrary, it is necessary to remember which will be used on each test port. \nParameters \n<cnum> Any existing channel number. If unspecified, value is set to 1 \n<conn1> Adapter port 1 connector type. Use SENS:CORR:COLL:GUID:CONN:CAT? \nto return a list of valid connector types. \n<conn2> Adapter port 2 connector type. \nExamples See example using this command. \nReturn Type Numeric \n1643\n\nDefault Not Applicable \nSENSe<cnum>:CORRection:COLLect:GUIDed:ADAPter:COUNt? \n(Read-Only) Returns the number of THRU adapters that have been created for this calibration using \nSENS:CORR:COLL:GUID:ADAP:CREate? \nParameters \n<cnum> Any existing channel number. If unspecified, value is set to 1 \nExamples See example using this command. \nReturn Type Numeric \nDefault Not Applicable \nSENSe<cnum>:CORRection:COLLect:GUIDed:ADAPter<n>:DELay <coax>, [w phase, \nwdelay] \n(Write-only) Specifies the adapter delay. and optionally waveguide delay and optional phase offset \n(degrees) of adapter <n>. \nParameters \n<cnum> Any existing channel number. If unspecified, value is set to 1 \n<n> Adapter index number that was returned from \nSENS:CORR:COLL:GUID:ADAP:CREate? \n<coax> Delay value of coax adapter <n> in seconds. If the adapter has no coax \nconnector, enter 0. \n<wphase> Waveguide phase offset in degrees. If the adapter has no waveguide connector, \ndo not enter a value. \n<wdelay> Waveguide delay in seconds. If the adapter has no waveguide connector, do not \nenter a value. \nExamples See example using this command. \nDefault Not Applicable \nSENSe<cnum>:CORRection:COLLect:GUIDed:ADAPter<n>:DESCription <string> \n1644\n\n(Write-only) Specifies the adapter description for use as the guided cal connection prompts. \nParameters \n<cnum> Any existing channel number. If unspecified, value is set to 1 \n<n> Adapter index number that was returned from \nSENS:CORR:COLL:GUID:ADAP:CREate? \n<string> Adapter description. \nExamples See example using this command. \nQuery Syntax Not Applicable \nDefault Not Applicable \nSENSe<cnum>:CORRection:COLLect:GUIDed:ADAPter<n>PATHs <port pairs> \n(Write-only) Specifies the port pairs for which the adapter will be used for a THRU connection. \nFor example, for a 3-port cal on channel 1 using ports 1,2,and 3), to use adapter 1 between the ports (1 \nto 2) and (1 to 3) the following command is used: SENS1:CORR:COLL:GUID:ADAP1:PATH \n1,2,1,3. \nThe adapter must have the same DUT connectors as the ports that are already specified for these ports. \nParameters \n<cnum> Any existing channel number. If unspecified, value is set to 1 \n<n> Adapter index number that was returned from \nSENS:CORR:COLL:GUID:ADAP:CREate? \n<port pair> Ports for which the adapter will be used. The orientation is not critical, as the \nPNA will align the connector types as necessary. The minimum number of \nThru connections required is the number of ports to calibrated -1. \nExamples See example using this command. \nQuery Syntax Not Applicable \nDefault Not Applicable \nSENSe:CORRection:COLLect:GUIDed:CKIT:PORT<pnum>:CATalog? \n1645\n\n(Read-only) Returns a comma-separated list of valid kits for each port. In addition to mechanical \ncalibration kits, this will include applicable characterizations found within ECal modules currently \nconnected to the PNA. \nIf two or more identical ECal modules are connected to the PNA, the returned list will include the \nserial numbers to distinguish the ECal modules. \nUse items in the list to select the kit to be used with the SENS:CORR:COLL:GUID:CKIT:PORT \ncommand. \nParameters \n<pnum> Any existing port number. If unspecified, value is set to 1 \nExamples SENS:CORR:COLL:GUID:CKIT:PORT1:CAT? \n'When \"Type N (50) male\" is specified for connector type, \nreturns: \n\"85054D, 85032F\" \n'When two identical ECal modules are connected for the connector \ntype, \n'the return string includes serial numbers \n\"85092-60010 ECal 10675, 85092-60010 ECal 00758\" \nReturn Type String \nDefault Not Applicable \nSENSe:CORRection:COLLect:GUIDed:CKIT:PORT<pnum>[:SELect] <kit> \n(Read-Write) Specifies the calibration kit for each port to be used during a guided calibration. An \nunused port does NOT need to have a specified Cal Kit. \nIf two or more identical ECal modules are connected to the PNA, the serial number must be included \nin the <kit> string to distinguish the ECal modules. See \nSENS:CORR:COLL:GUID:CKIT:PORT:CAT? \nNote: Sliding loads are not fully supported from Sens:Corr:Coll:Guided... The Measure button must \nbe manually pressed. \n1. Specify the connector type for the port with SENS:CORR:COLL:GUID:CONN:PORT. \n2. Query the valid available kits for the connector on each port with \nSENS:CORR:COLL:GUID:CKIT:PORT:CAT? \n1646\n\n3. Specify the kit using this command. \n4. Perform a query of this command. If the <kit> parameter was incorrectly entered, an error will be \nreturned.\nParameters \n<pnum> Any existing port number. If unspecified, value is set to 1 \n<kit> Calibration kit to be used for the specified port. \nExamples SENS:CORR:COLL:GUID:CKIT:PORT1 '85055A' \n'The following includes a serial number when two or more ECal \nmods are connected \nsense:correction:collect:guided:ckit:port2:select '85092-60010 \nECal 10685' \nQuery Syntax SENSe:CORRection:COLLect:GUIDed:CKIT:PORT<pnum>[:SELect]? \nReturn Type String - If the <kit> parameter was incorrectly entered while writing, an error \nwill be returned. \nDefault Not Applicable \nSENSe:CORRection:COLLect:GUIDed:CONNector:CATalog? \n(Read only) Returns a list of valid connectors based on the connector descriptions of the available cal \nkits. Use an item from the returned list to specify a connector for \nSENS:CORR:COLL:GUID:CONN:PORT \nExamples SENS:CORR:COLL:GUID:CONN:CAT? \nReturns: \nType N (50) female, Type N (50) male, APC 7 (50), 3.5 mm (50) \nmale, 3.5 mm (50) female, User Connector A \nReturn Type Comma separated string values \nDefault Not Applicable \nSENSe:CORRection:COLLect:GUIDed:CONNector:PORT<pnum>[:SELect] <conn> \n1647\n\n(Read-Write) Specifies a connector type for every port during the Guided Calibration procedure. Valid \nconnector names are stored within calibration kits. Some cal kits may include both male and female \nconnectors. Therefore, specifying connector gender may be required. \nThe PNA remembers previous Guided Cal settings. Therefore, for completeness, unused ports should \nbe defined as \"Not used\". See Guided Cal examples. \nA single port with a valid <conn> name indicates a 1-Port calibration will be performed. \nTwo ports with valid <conn> names indicate either a 2-Port SOLT or TRL calibration will be performed \ndepending on the standards definition found within the cal kit and the capability of the PNA. \nThree ports with valid <conn> names indicate a 3-Port calibration will be performed, and so forth. \nThe following steps could be followed to ensure port connectors are specified correctly: \nUse SENS:CORR:COLL:GUID:CONN:CAT? to query available connectors before specifying the port \nconnector. \n1. \nSelect a connector type using this command. 2. \nPerform a query of this command. If the <conn> parameter was incorrectly entered, an error will be \nreturned. \n3. \nSpecify the cal kit to use for each port with SENS:CORR:COLL:GUID:CKIT:PORT 4. \nParameters \n<pnum> Any existing port number. If unspecified, value is set to 1 \n<conn> String - DUT connector type to connect with PNA port <pnum> \nExamples 'Specifying a 2-port cal (1 & 2) on a 4-port PNA \nSENS:CORR:COLL:GUID:CONN:PORT1 'Type N (50) female' \nSENS:CORR:COLL:GUID:CONN:PORT2 'Type N (50) male' \nSENS:CORR:COLL:GUID:CONN:PORT3 'Not Used' \nSENS:CORR:COLL:GUID:CONN:PORT4 'Not Used' \nQuery Syntax SENSe:CORRection:COLLect:GUIDed:CONNector:PORT<pnum>[:SELect]? \nReturn Type String \nDefault Not Applicable \nSENSe:CORRection:COLLect:GUIDed:DESCription? <step> \n1648\n\n(Read-only) Returns the connection description for the specified calibration step. \nParameters \n<step> A number from 1 to the number of steps required to complete the calibration \n(Use SENS:CORR:COLL:GUID:STEP? to query the number of steps ) \nExamples SENS:CORR:COLL:GUID:DESC? 10 \n'Returns: \nConnect APC 7 Open to port3 \nReturn Type String \nDefault Not Applicable \nSENSe:CORRection:COLLect:GUIDed:DMATch:APPLy[:IMMediate] [<CalSetGUID>] \n(Write-only) Specifies a Cal Set as a source of delta match correction. \nIf CalSetGUID is not specified, then the Global Delta Match Cal Set is assumed. An error is returned \nif the specified Cal Set does not meet the following Delta Match criteria. The Global Delta Match Cal \ncan ALWAYS be applied. \nMust have been performed using ECal or as a guided mechanical cal (not Unguided). \nMust have the same start freq, stop freq, and number of points as the channel being calibrated. \nMust calibrate the ports that are required by the TRL or Unknown Thru cal as indicated by \nSENS:CORR:COLL:GUID:DMATch:APPLy:PORTs?. \nLearn more about Delta match calibration. \nSee example of a complete Delta Match calibration. \nParameters \n<CalSetGUID> Optional. GUID of the Cal Set to use. If unspecified, the Global Delta Match \nCal Set is used. \nExamples SENS:CORR:COLL:GUID:DMAT:APPL \nsense:correction:collect:guided:dmatch:apply:immediate \n\"{2B893E7A-971A-11d5-8
